vi "Update Generation on the Fly.vi"(8 "error in (no error)":errorcluster, 9 "output level units":T1, 10 "sine wave properties":T2, 11 "Digital Serial in":refnum<class "Digital Serial.lvclass">) -> (0 "error out":errorcluster, 3 "Digital Serial out":refnum<class "Digital Serial.lvclass">)   [LabVIEW 2023, in "Digital Serial.lvclass"]
uses:
  Digital Serial.lvclass
  service/generation/controls/sine wave properties.ctl
  controls/digital output level units.ctl
  Digital Serial.lvclass/Digital Serial.ctl
  <vilib>/PDM Acquisition Toolkit/host/Classes/Channels/PCM Output/PCM Output Channel.lvclass
  C:/Program Files/NI/LVAddons/pdm/1/vi.lib/PDM Acquisition Toolkit/host/Classes/Channels/DecoderChannel.lvclass
  <vilib>/PDM Acquisition Toolkit/host/Classes/Channels/PCM Output/controls/PCM Output Channel - Signal Properties.ctl
  <vilib>/PDM Acquisition Toolkit/host/Classes/Tasks/PCM Output/PCM Output Task.lvclass
  C:/Program Files/NI/LVAddons/pdm/1/vi.lib/PDM Acquisition Toolkit/host/Classes/Tasks/Parent/DecoderTask.lvclass
  <vilib>/PDM Acquisition Toolkit/host/Classes/Channels/DecoderChannel.lvclass
  service/generation/controls/AudioGenTypeDefs.lvlib
  controls/audio controls.lvlib
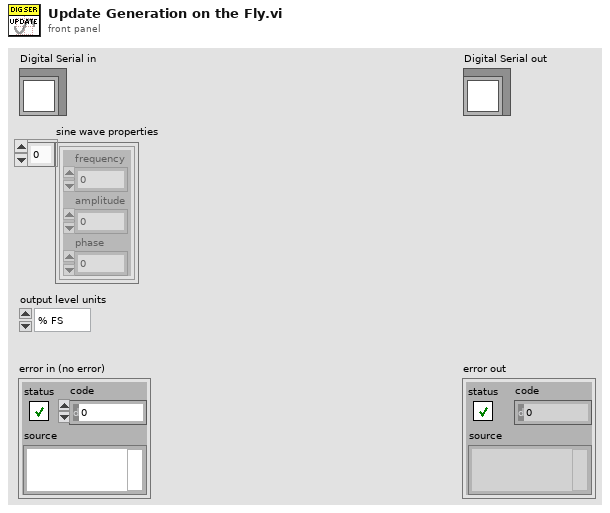
[diagram p1: front panel]
types:
  T1 = typedef "audio controls.lvlib/digital output level units.ctl" = enum32{"% FS", "dBFS", "V"}
  T2 = typedef "AudioGenTypeDefs.lvlib/sine wave properties.ctl" = cluster{"frequency":dbl, "amplitude":dbl, "phase":dbl}[]
  T3 = typedef "PDM Acquisition Class Library.lvlib/PCM Output Task.lvclass/PCM Output Task DVR.ctl" = refnum<data-value>
  T4 = typedef "PDM Acquisition Class Library.lvlib/PCM Output Channel.lvclass/PCM Output Channel - Signal Properties.ctl" = cluster{"cyclic period":dbl, "cyclic phase offset":dbl, "gain":dbl}
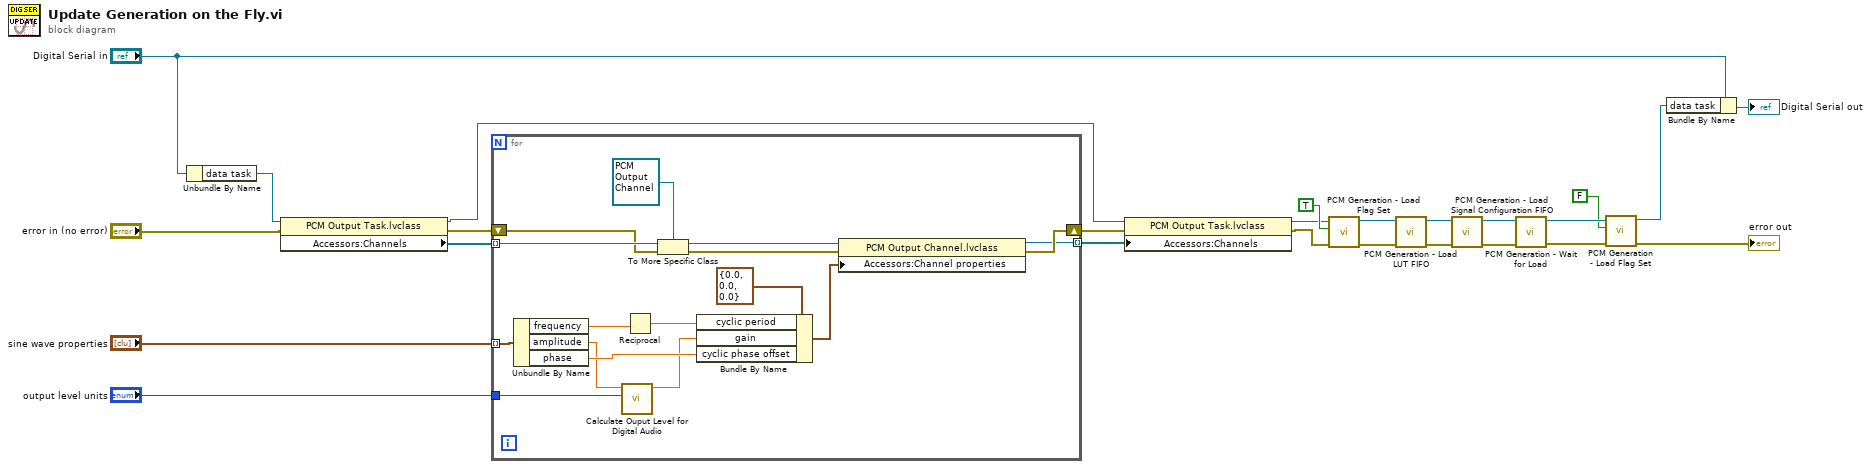
[diagram p0: block diagram]
diagram:
  n1 = Unbundle By Name("Digital Serial in") -> ("data task"=w4:T3)
  n2 = property class="PCM Output Task.lvclass"(reference=w4, error in="error in (no error)") -> (reference out=w12:T3, error out=w24:errorcluster, "Accessors:Channels"=w25:refnum<class "DecoderChannel.lvclass">[])
  n3 = for {
    tunnel: w25 -> [w40] mode=indexing
    shift-right: [w36] -> w14
    shift-left: w24 -> [w38]
    tunnel: [w35] -> w13 mode=indexing
    tunnel: "sine wave properties" -> [w31] mode=indexing
    tunnel: "output level units" -> [w26]
    n4 = Unbundle By Name(w31) -> ("frequency"=w30:dbl, "amplitude"=w28:dbl, "phase"=w29:dbl)
    n5 = call "Calculate Ouput Level for Digital Audio.vi"("digital output level units"=w26, "output level"=w28) -> ("gain"=w27:dbl)  [unwired: 8 in, 1 out]
    n6 = Reciprocal(x=w30) -> (1/x=w34:dbl)
    n7 = To More Specific Class(target class=refnum<class "PCM Output Channel.lvclass"> refnum ("PDM Acquisition Class Library.lvlib:PCM Output Channel.lvclass"), reference=w40, error in=w38) -> (specific class reference=w37:refnum<class "PCM Output Channel.lvclass">, error out=w41:errorcluster)
    n8 = Bundle By Name(cluster=T4 {"cyclic period"=0.0, "cyclic phase offset"=0.0, "gain"=0.0} ("Channel properties"), "cyclic period"=w34, "gain"=w27, "cyclic phase offset"=w29) -> (w32:T4)
    n9 = property class="PCM Output Channel.lvclass"(reference=w37, error in=w41, "Accessors:Channel properties"=w32) -> (reference out=w35:refnum<class "PCM Output Channel.lvclass">, error out=w36:errorcluster)
  }
  n10 = property class="PCM Output Task.lvclass"(reference=w12, error in=w14, "Accessors:Channels"=w13) -> (reference out=w11:T3, error out=w10:errorcluster)
  n11 = call <vilib>:"PCM Generation - Load Flag Set.vi"("error in"=w10, "Load"=TRUE, "PCM Output Task In"=w11) -> ("error out"=w18:errorcluster, "PCM Output Task Out"=w17:T3)  [unwired: 7 in]
  n12 = call <vilib>:"PCM Generation - Load LUT FIFO.vi"("error in"=w18, "PCM Output Task In"=w17) -> ("error out"=w15:errorcluster, "PCM Output Task Out"=w16:T3)  [unwired: 8 in]
  n13 = call <vilib>:"PCM Generation - Load Signal Configuration FIFO.vi"("error in"=w15, "PCM Output Task In"=w16) -> ("error out"=w9:errorcluster, "PCM Output Task Out"=w19:T3)  [unwired: 8 in]
  n14 = call <vilib>:"PCM Generation - Wait for Load.vi"("error in"=w9, "PCM Output Task In"=w19) -> ("error out"=w21:errorcluster, "PCM Output Task Out"=w22:T3)  [unwired: 7 in, 1 out]
  n15 = call <vilib>:"PCM Generation - Load Flag Set.vi"("error in"=w21, "Load"=FALSE, "PCM Output Task In"=w22) -> ("error out"=→"error out":errorcluster, "PCM Output Task Out"=w2:T3)  [unwired: 7 in]
  n16 = Bundle By Name(cluster="Digital Serial in", "data task"=w2) -> (→"Digital Serial out":refnum<class "Digital Serial.lvclass">)
